vi "getOutputStateArray.vi"(8 "error in (no error)":errorcluster, 11 "OutputConfiguration in":refnum<class "OutputConfiguration.lvclass">) -> (0 "error out":errorcluster, 2 "outputStateArray":cluster{"channel":string, "state":string}[](array[cluster]), 3 "OutputConfiguration out":refnum<class "OutputConfiguration.lvclass">)   [LabVIEW 2011, in "Tools.lvlib" / "DatabaseHelpers.lvlib" / "OutputConfiguration.lvclass"]
uses:
  OutputConfiguration.lvclass
  OutputConfiguration.lvclass/OutputConfiguration.ctl
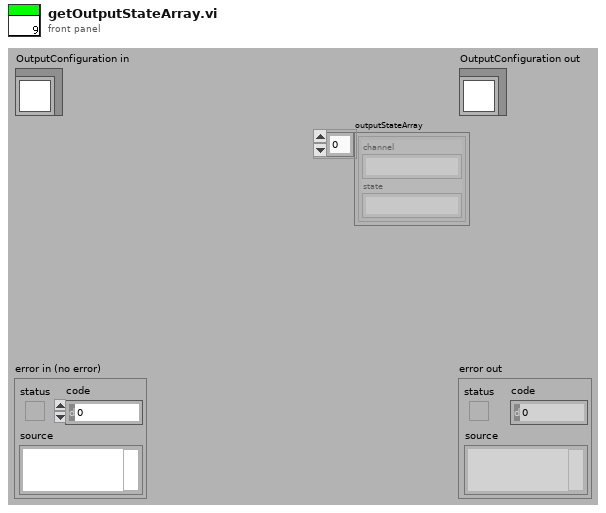
[diagram p1: front panel]
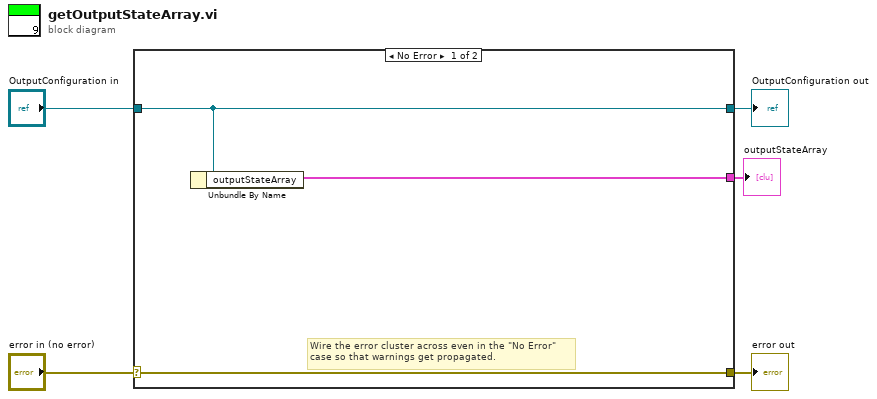
[diagram p0: block diagram]
diagram:
  n1 = case shown="No Error" "error in (no error)" {
    selector: "error in (no error)" -> [w8 w10]
    tunnel: [w8 w10] -> w4
    tunnel: [w7 w9] -> w2
    tunnel: "OutputConfiguration in" -> [w7 w9]
    tunnel: [w6 _] -> w1
    frame No Error {
      # "Wire the error cluster across even in the \"No Error\"\ncase so that warnings get propagated."
      n2 = Unbundle By Name(w7) -> ("outputStateArray"=w6:cluster{"channel":string, "state":string}[])
    }
    frame Error {
    }
  }
  "error out" <- w4
  "OutputConfiguration out" <- w2
  "outputStateArray" <- w1
